vi "RSZVB Option Checking.vi"(8 "error in (no error)":errorcluster {"code" format="%.0x"}, 10 "Option Checking (T: On)":bool=TRUE, 11 "VISA session":refnum<visa-resource-name>) -> (0 "error out":errorcluster {"code" format="%.0x"}, 3 "dup VISA session":refnum<visa-resource-name>)   [LabVIEW 2011]
doc: "This VI switches option checking of the instrument."
uses:
  _utility/RSZVB Global Data.vi
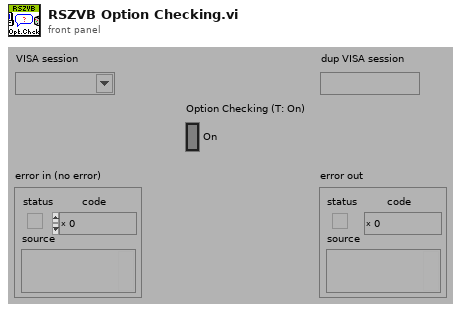
[diagram p1: front panel]
types:
  T1 = cluster{"Error Checking (T: On)":bool, "Installed Options":string[], "Data Valid?":bool, "Ports":i32, "Model":string[], "Option Checking (T: On)":bool}[]
  T2 = cluster{"Error Checking (T: On)":bool, "Installed Options":string[], "Data Valid?":bool, "Ports":i32, "Model":string[], "Option Checking (T: On)":bool}
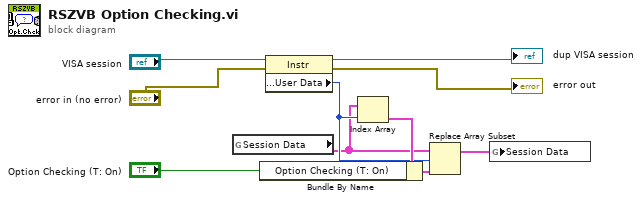
[diagram p0: block diagram]
diagram:
  n1 = global read "RSZVB Global Data.vi" "Session Data"() -> (w7:T1)
  n2 = property class="Instr"(reference="VISA session", error in="error in (no error)") -> (reference out=→"dup VISA session":refnum<visa-resource-name>, error out=→"error out":errorcluster, "General Settings:User Data"=w9:u32)
  n3 = Index Array(array=w7, index=w9) -> (element=w10:T2)
  n4 = Bundle By Name(cluster=w10, "Option Checking (T: On)"="Option Checking (T: On)") -> (w8:T2)
  n5 = Replace Array Subset(array=w7, new element=w8, index=w9) -> (w6:T1)
  n6 = global write "RSZVB Global Data.vi" "Session Data"(w6) -> ()
